vi "DelChanCurveRef.vi"(8 "错误输入（无错误）":errorcluster, 11 "曲线参考点索引":u8) -> (0 "错误输出":errorcluster)   [LabVIEW 2014]
uses:
  X86Dll/ZXUTConfigMgr.dll
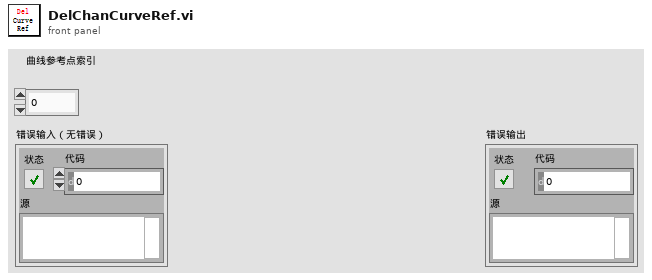
[diagram p1: front panel]
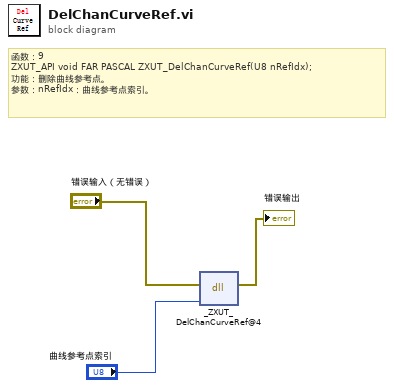
[diagram p0: block diagram]
diagram:
  # "函数：9\nZXUT_API void\tFAR PASCAL ZXUT_DelChanCurveRef(U8 nRefIdx);\n功能：删除曲线参考点。\n参数：nRefIdx：曲线参考点索引。"
  n1 = dll-call lib="D:/Software/Utrasonic on-line monitoring/X86Dll/ZXUTConfigMgr.dll" fn="_ZXUT_DelChanCurveRef@4"(error in="错误输入（无错误）", "nRefIdx"="曲线参考点索引") -> (error out=→"错误输出":errorcluster)  [unwired: 4 in, 1 out]
